vi "Transmit I32 Data.vi"(8 "error in (no error)":errorcluster, 10 "Data":i32[](array[numeric]), 11 "RP Communicator in":refnum<class "RP Communicator.lvclass">) -> (0 "error out":errorcluster, 3 "RP Communicator out":refnum<class "RP Communicator.lvclass">)   [LabVIEW 2019, in "RP Communicator.lvclass"]
uses:
  RP Communicator.lvclass
  RP Communicator.lvclass/RP Communicator.ctl
  RP Transmit Data TCP.vi
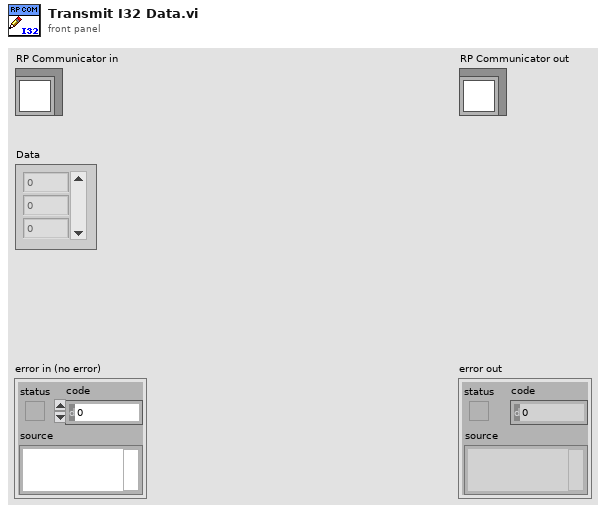
[diagram p1: front panel]
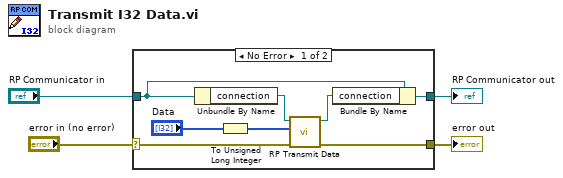
[diagram p0: block diagram]
diagram:
  n1 = case shown="No Error" "error in (no error)" {
    selector: "error in (no error)" -> [w8 w14]
    tunnel: [w7 w14] -> w3
    tunnel: [w6 w13] -> w1
    tunnel: "RP Communicator in" -> [w12 w13]
    frame No Error {
      n2 = Unbundle By Name(w12) -> ("connection"=w11:refnum<k5>)
      n3 = To Unsigned Long Integer(number="Data") -> (unsigned 32bit integer=w9:u32[])
      n4 = call-poly "RP Transmit Data.vi"("Error In"=w8, "Data"=w9, "connection ID"=w11) -> ("Error Out"=w7:errorcluster, "connection ID out"=w5:refnum<k5>)  [unwired: 7 in]
      n5 = Bundle By Name(cluster=w12, "connection"=w5) -> (w6:refnum<class "RP Communicator.lvclass">)
    }
    frame Error {
    }
  }
  "error out" <- w3
  "RP Communicator out" <- w1
